vi "Contiguous Structure Converter Assistant.vi"(8 "error in (no error)":errorcluster, 10 "Original JSON":string, 11 "Contiguous Structure from JSON Parse":T5) -> (0 "error out":errorcluster, 3 "Contiguous Structure":T1)   [LabVIEW 2021, in "DataTypes_CIF_U.lvlib"]
doc: "This helper utility should be used with a JSON parse VI. The Contiguous Structure from JSON Parse should be the input type for parsing a JSON created from the \"Get JSON Descriptor of Variant\" VI and can be used as an interface description for a contigous data element (primative, cluster, or 1D array of fixed size). The JSON parse is not included to allow flexibility on using various parsers."
uses:
  DataTypes_CIF_U.lvlib
  Typedef/Endian.ctl
  Typedef/Generic Datatypes.ctl
  Typedef/Element.ctl
  Typedef/Contiguous Structure.ctl
  Typedef/Errors.ctl
  Typedef/Contiguous Structure for JSON Parse.ctl
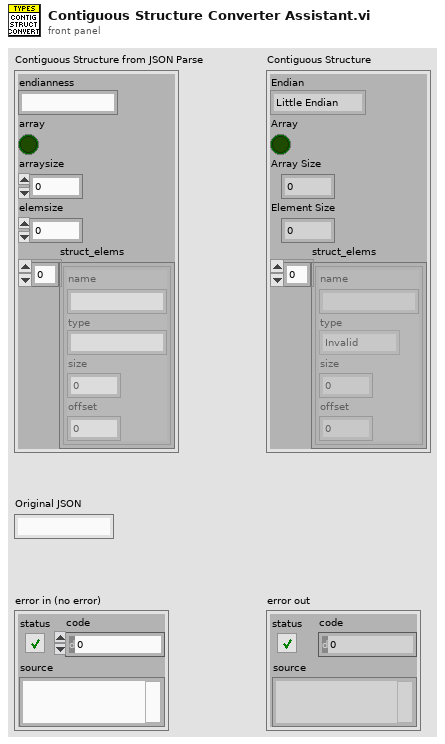
[diagram p1: front panel]
types:
  T1 = typedef "DataTypes_CIF_U.lvlib/Contiguous Structure.ctl" = cluster{"Endian":T2, "Array":bool, "Array Size":u32, "Element Size":u32, "struct_elems":T3[]}
  T2 = typedef "DataTypes_CIF_U.lvlib/Endian.ctl" = enum16{"Little Endian", "Big Endian"}
  T3 = typedef "Element.ctl" = cluster{"name":string, "type":T4, "size":u32, "offset":u32}
  T4 = typedef "DataTypes_CIF_U.lvlib/Generic Datatypes.ctl" = enum16{"Invalid", "Bool", "U8", "I8", "U16", "I16", "U32", "I32", "U64", "I64", "Single Float", "Double Float", "String"}
  T5 = typedef "DataTypes_CIF_U.lvlib/Contiguous Structure for JSON Parse.ctl" = cluster{"endianness":string, "array":bool, "arraysize":u32, "elemsize":u32, "struct_elems":cluster{"name":string, "type":string, "size":u32, "offset":u32}[]}
  T6 = typedef "DataTypes_CIF_U.lvlib/Errors.ctl" = enum16{"Too few bytes", "Unsupported Type", "Invalid GUID", "Error Parsing JSON"}
  T7 = cluster{"name":string, "type":string, "size":u32, "offset":u32}[]
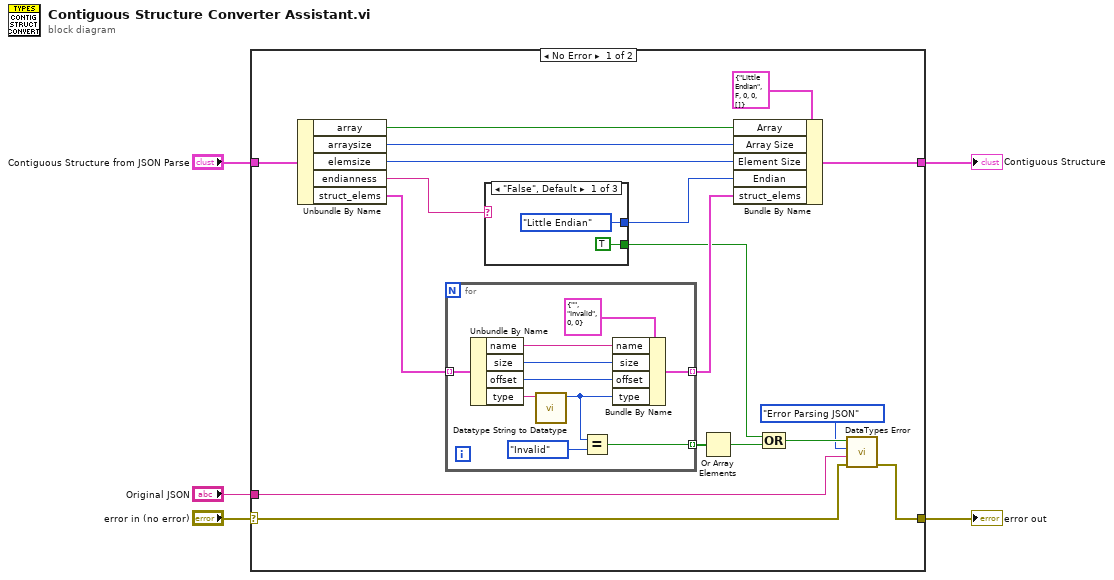
[diagram p0: block diagram]
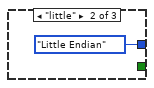
[diagram p2: hidden frame]
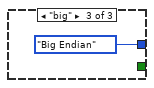
[diagram p3: hidden frame]
diagram:
  n1 = case shown="No Error" "error in (no error)" {
    selector: "error in (no error)" -> [w6 w38]
    tunnel: [w19 _] -> w5
    tunnel: "Contiguous Structure from JSON Parse" -> [w9 _]
    tunnel: "Original JSON" -> [w8 _]
    tunnel: [w7 w38] -> w2
    frame No Error {
      n2 = Unbundle By Name(w9) -> ("array"=w22:bool, "arraysize"=w21:u32, "elemsize"=w20:u32, "endianness"=w16:string, "struct_elems"=w18:T7)
      n3 = for {
        tunnel: w18 -> [w37] mode=indexing
        tunnel: [w32] -> w17 mode=indexing
        tunnel: [w28] -> w14 mode=indexing
        n4 = Unbundle By Name(w37) -> ("name"=w35:string, "size"=w34:u32, "offset"=w33:u32, "type"=w31:string)
        n5 = call "Datatype String to Datatype.vi"("Datatype String"=w31) -> ("Generic Datatype"=w29:T4)  [unwired: 10 in]
        n6 = Equal?(x=w29, y=Generic_Datatypes."Invalid" ("type")) -> (x = y?=w28:bool)
        n7 = Bundle By Name(cluster=T3 {"name"="", "type"=enum."Invalid", "size"=0, "offset"=0} ("Element"), "name"=w35, "size"=w34, "offset"=w33, "type"=w29) -> (w32:T3)
      }
      n8 = case shown="\"False\", Default" w16 {
        tunnel: [Endian."Little Endian" ("Endian") Endian."Little Endian" ("Endian") Endian."Big Endian" ("Endian")] -> w15
        tunnel: [TRUE _ _] -> w13
        frame "False", Default {
        }
        frame "little" {
        }
        frame "big" {
        }
      }
      n9 = Or Array Elements(Boolean array=w14) -> (logical OR=w12:bool)
      n10 = Bundle By Name(cluster=T1 {"Endian"=enum."Little Endian", "Array"=FALSE, "Array Size"=0, "Element Size"=0, "struct_elems"=[]} ("Contiguous Structure 2"), "Array"=w22, "Array Size"=w21, "Element Size"=w20, "Endian"=w15, "struct_elems"=w17) -> (w19:T1)
      n11 = Compound Arithmetic op=OR(w13, w12) -> (w11:bool)
      n12 = call "DataTypes Error.vi"("error in (no error)"=w6, "String to Append"=w8, "Error"=Errors."Error Parsing JSON", "Insert Error"=w11) -> ("error out"=w7:errorcluster)  [unwired: 7 in]
    }
    frame Error {
    }
  }
  "Contiguous Structure" <- w5
  "error out" <- w2
